vi "ROSServiceProvider.vi"(2 "Response":T2, 3 "ROS":T3={"topic port"=1236, "Node"="/labview", "topic"="/robot/head/command_head_nod", "type"="std_msgs/Bool", "node port"=7000, "error "={"status"=FALSE, "code"=0, "source"=""}, "Direction"=enum."Publisher", "Update (ms)"=1, "FIFO size"=1}) -> ()   [LabVIEW 2015]
doc: "Opens new ports for services, updates services with master, and closes services"
uses:
  SubVIs/_ROSControl.ctl
  SubVIs/_ROSDirection.ctl
  Console/Servers/ServerSubs/MyState.ctl
  _ROSDefinition.vi
  MessageBuilding/std_msgs/subs/i16Scalar.vi
  MessageBuilding/std_msgs/subs/stringScalar.vi
panel:
  out "Queue":string
  out "Master Reply":T1(array[cluster])
  out "response":string
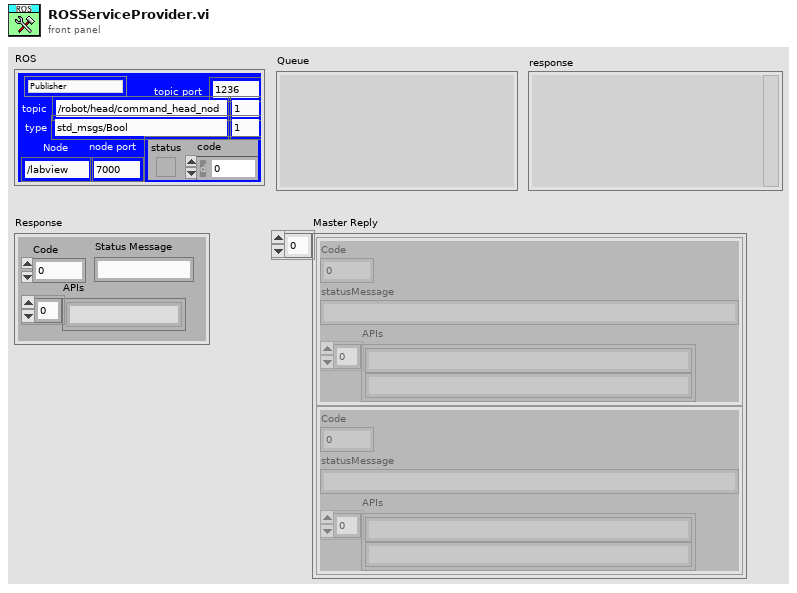
[diagram p1: front panel]
types:
  T1 = cluster{"Code":i8, "statusMessage":string, "APIs":string[]}[]
  T2 = cluster{"Code":i32, "Status Message":string, "APIs":string[]}
  T3 = typedef "_ROSControl.ctl" = cluster{"topic port":u16, "Node":string, "topic":string, "type":string, "node port":u16, "error ":errorcluster, "Direction":T4, "Update (ms)":u16, "FIFO size":u16}
  T4 = typedef "_ROSDirection.ctl" = enum16{"Node", "Publisher", "Subscriber", "ServiceClient", "ServiceProvider"}
  T5 = typedef "MyState.ctl" = enum16{"No Connection", "Registered", "Connected", "Close"}
  T6 = enum16{"Reset Log", "Add Client", "Remove Client", "Add Task"}
  T7 = typedef "ROSLog.ctl" = cluster{"Sent":string, "Reply":string, "MethodName":string, "success":bool, "Dir1":string, "Dir2":string, "Time Stamp":string, "error":errorcluster, "Preamble":string, "Midamble":string, "Postamble":string}
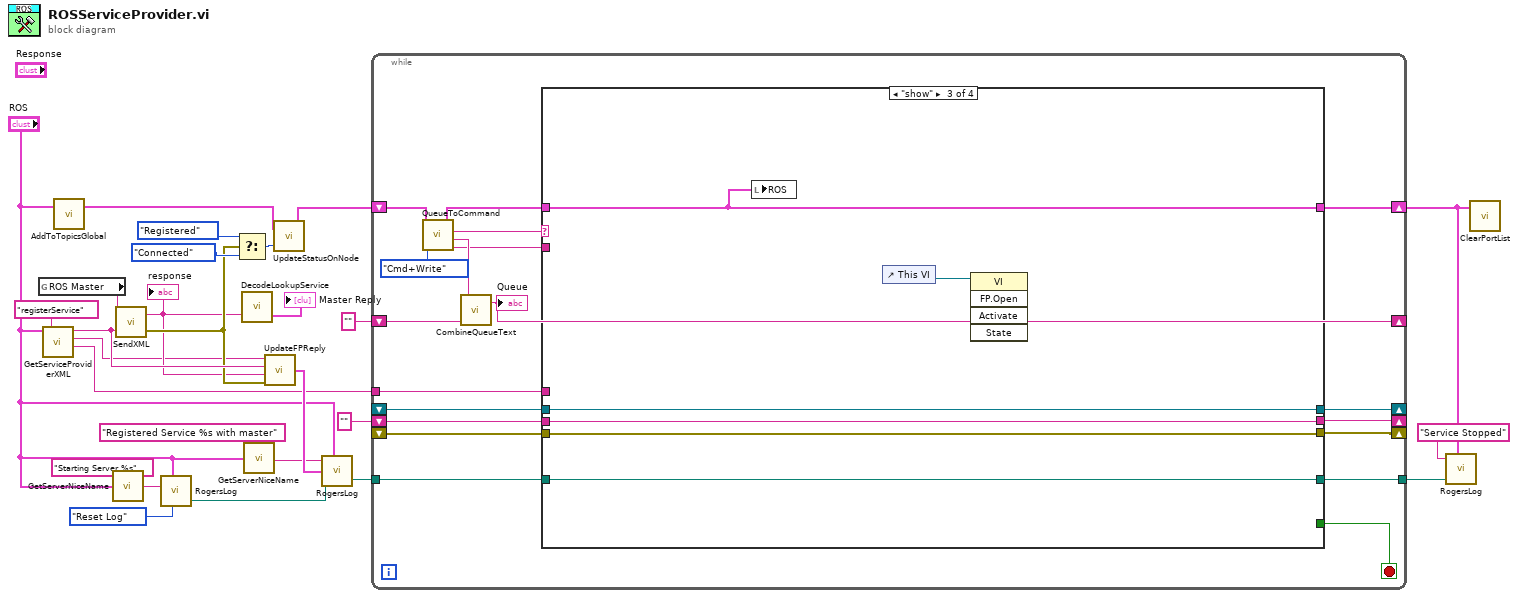
[diagram p0: block diagram]
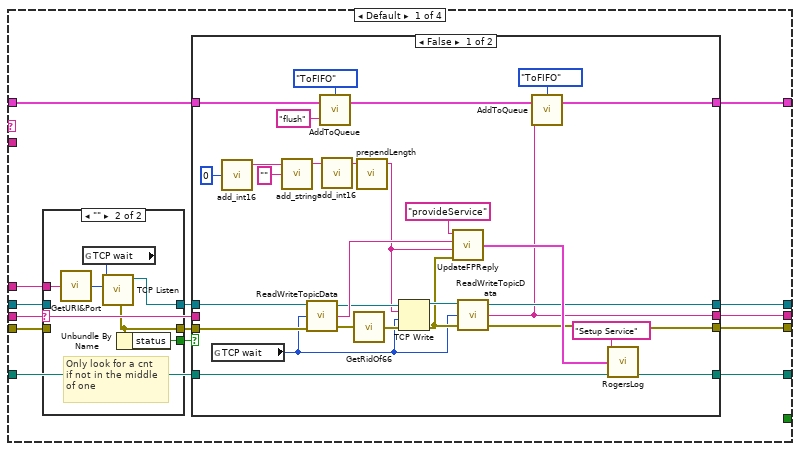
[diagram p2: hidden frame]
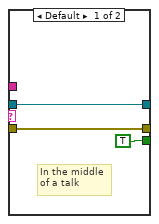
[diagram p3: hidden frame]
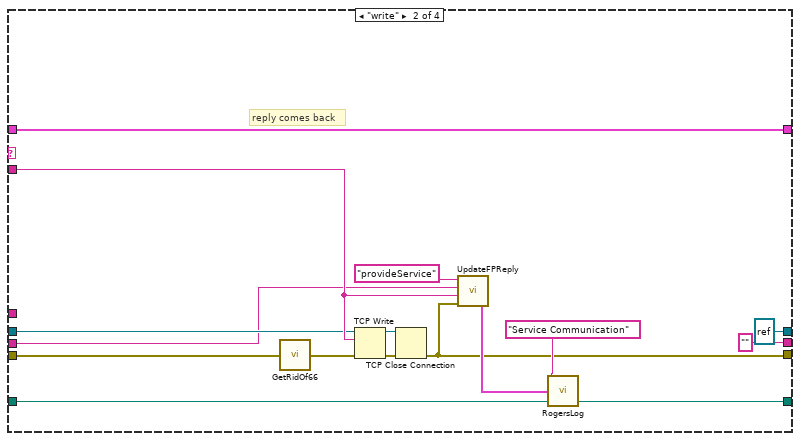
[diagram p5: hidden frame]
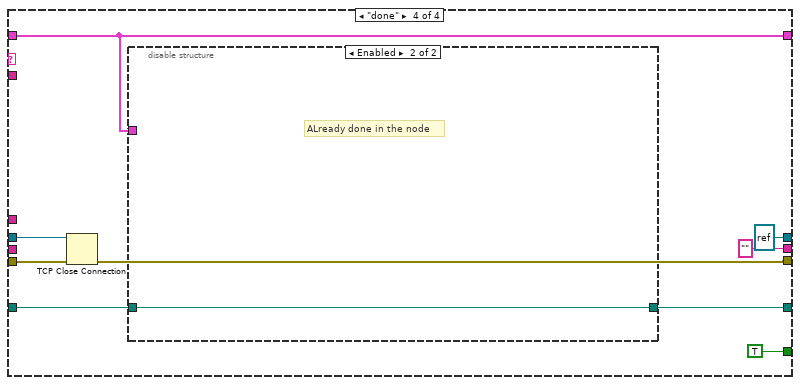
[diagram p6: hidden frame]
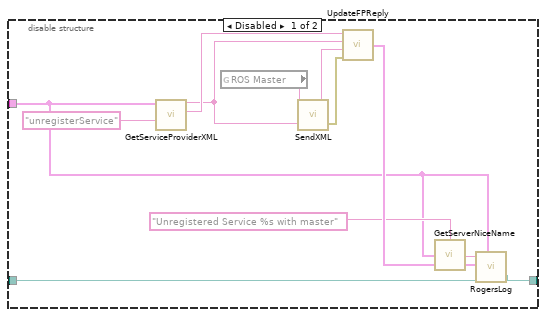
[diagram p7: hidden frame]
diagram:
  n1 = global read "_ROSDefinition.vi" "ROS Master"() -> (w23:string)
  n2 = call "GetServiceProviderXML.vi"("Method Name"="registerService", "ROS"="ROS") -> ("URI"=w6:string, "Method Name"=w9:string, "lookupService"=w24:string)  [unwired: 7 in]
  n3 = call "AddToTopicsGlobal.vi"("ROS in"="ROS") -> ("ROS out"=w3:T3)  [unwired: 2 in]
  n4 = call "GetServerNiceName.vi"("ROS"="ROS", "Text to add"="Starting Server %s") -> ("String"=w26:string)
  n5 = call "SendXML.vi"("Send"=w24, "URI in"=w23) -> ("error out"=w15:errorcluster, "Reply"=w14:string)
  "response" <- w14
  n6 = call "RogersLog.vi"("Text to add"=w26, "ROS"="ROS", "Task"=T6."Reset Log") -> ("LogPath out"=w18:path)  [unwired: 2 in, 1 out]
  n7 = Select(t=MyState."Registered" ("MyState"), s=w15, f=MyState."Connected" ("MyState")) -> (s? t:f=w20:T5)
  n8 = call "DecodeLookupService.vi"("Response"=w14) -> ("Reply"=→"Master Reply":T1)  [unwired: 2 in]
  n9 = call "GetServerNiceName.vi"("ROS"="ROS", "Text to add"="Registered Service %s with master") -> ("String"=w16:string)
  n10 = call "UpdateFPReply.vi"("error in (no error)"=w15, "Reply"=w14, "Sent"=w24, "method"=w9) -> ("Log"=w19:T7)
  n11 = call "UpdateStatusOnNode.vi"("MyState"=w20, "ROS"=w3) -> ("ROS out"=w2:T3)  [unwired: 1 in]
  n12 = call "RogersLog.vi"("Text to add"=w16, "ROS"="ROS", "Log"=w19, "LogPath in"=w18) -> ("LogPath out"=w11:path)  [unwired: 1 in, 1 out]
  n13 = while {
    tunnel: w11 -> [w46]
    tunnel: [w45] -> w10
    shift-right: [w41] -> _
    shift-left: "" ("New List") -> [w42]
    tunnel: w6 -> [w40]
    shift-right: [w36] -> _
    shift-left: _ -> [w33]
    shift-right: [w35] -> _
    shift-left: "" ("data out") -> [w31]
    shift-right: [w34] -> _
    shift-left: _ -> [w32]
    shift-right: [w29] -> w1
    shift-left: w2 -> [w39]
    stop <- w44 stop-if-true
    n14 = call "QueueToCommand.vi"("ROS"=w39, "Check"=enum16{"Cmd+Write", "FIFO", "CMD", "CMD /wait"}."Cmd+Write") -> ("ROS out"=w30:T3, "Command"=w38:string, "Queue log"=w43:string, "data"=w37:string)  [unwired: 1 in]
    n15 = call "CombineQueueText.vi"("Old List"=w42, "Queue In"=w43) -> ("New List"=w41:string)  [unwired: 1 in]
    "Queue" <- w41
    n16 = case shown="\"show\"" w38 {
      tunnel: w30 -> [w59 w106 w120 w133]
      tunnel: w46 -> [w58 w109 w125 w132]
      tunnel: [w57 w108 w125 w131] -> w45
      tunnel: w37 -> [_ w114 _ _]
      tunnel: [w47 w106 w120 w133] -> w29
      tunnel: [_ _ _ TRUE] -> w44
      tunnel: w40 -> [w56 _ _ _]
      tunnel: [w55 refnum<k5> refnum ("connection ID out") w121 refnum<k5> refnum ("connection ID out")] -> w36
      tunnel: [w54 "" ("data out") w122 "" ("data out")] -> w35
      tunnel: [w53 w107 w123 w128] -> w34
      tunnel: w33 -> [w50 w112 w121 w129]
      tunnel: w32 -> [w51 w111 w123 w130]
      tunnel: w31 -> [w52 w110 w122 _]
      frame Default {
        n17 = case shown="\"\"" w52 {
          tunnel: [w63 w65] -> w49
          tunnel: [w62 w68] -> w60
          tunnel: w56 -> [_ w66]
          tunnel: w51 -> [w63 _]
          tunnel: w50 -> [w62 _]
          tunnel: [TRUE w64] -> w48
          frame Default {
            # "In the middle\nof a talk"
          }
          frame "" {
            # "Only look for a cnt\nif not in the middle\nof one"
            n18 = call "GetURI&Port.vi"("URI in"=w66) -> ("Port"=w69:u16)  [unwired: 1 out]
            n19 = global read "_ROSDefinition.vi" "TCP wait"() -> (w67:i32)
            n20 = call "TCP Listen.vi"("timeout ms (wait forever: -1)"=w67, "port"=w69) -> ("error out"=w65:errorcluster, "connection ID"=w68:refnum<k5>)  [unwired: 5 in, 3 out]
            n21 = Unbundle By Name(w65) -> ("status"=w64:bool)
          }
        }
        n22 = case shown="False" w48 {
          tunnel: w60 -> [w98 w102]
          tunnel: w58 -> [w94 w103]
          tunnel: w59 -> [w73 w99]
          tunnel: [w77 w103] -> w57
          tunnel: [w80 w102] -> w55
          tunnel: [w79 w101] -> w54
          tunnel: [w78 w100] -> w53
          tunnel: w52 -> [_ w101]
          tunnel: w49 -> [w76 w100]
          tunnel: [w71 w99] -> w47
          frame False {
            n23 = global read "_ROSDefinition.vi" "TCP wait"() -> (w75:i32)
            n24 = call-poly "add_int16.vi"("Numeric"=i16 0) -> ("msg out"=w90:string)  [unwired: 4 in]
            n25 = call-poly "add_string.vi"("String"="", "msg in"=w90) -> ("msg out"=w91:string)  [unwired: 3 in]
            n26 = call "ReadWriteTopicData.vi"("error in (no error)"=w76, "timeout ms (1000)"=w75, "connection ID in"=w98) -> ("error out"=w97:errorcluster, "data out"=w96:string, "connection ID out"=w88:refnum<k5>)
            n27 = call "AddToQueue.vi"("Cmd"="flush", "ROS"=w73, "Type"=enum16{"topic", "node", "ToFIFO", "ToWrite"}."ToFIFO") -> ("ROS out"=w72:T3)  [unwired: 2 in]
            n28 = call-poly "add_int16.vi"("msg in"=w91) -> ("msg out"=w83:string)  [unwired: 4 in]
            n29 = call "GetRidOf66.vi"("error in (no error)"=w97) -> ("error out"=w89:errorcluster)
            n30 = call "prependLength.vi"("msg in"=w83) -> ("msg out"=w82:string)  [unwired: 4 in]
            n31 = TCP Write(connection ID=w88, data in=w82, error in (no error)=w89, 9:w75) -> (connection ID out=w87:refnum<k5>, error out=w86:errorcluster)  [unwired: 1 out]
            n32 = call "UpdateFPReply.vi"("error in (no error)"=w86, "Reply"=w82, "Sent"=w96, "method"="provideService") -> ("Log"=w85:T7)
            n33 = call "ReadWriteTopicData.vi"("error in (no error)"=w86, "timeout ms (1000)"=w75, "connection ID in"=w87) -> ("error out"=w78:errorcluster, "data out"=w79:string, "connection ID out"=w80:refnum<k5>)
            n34 = call "AddToQueue.vi"("Cmd"=w79, "ROS"=w72, "Type"=enum16{"topic", "node", "ToFIFO"}."ToFIFO") -> ("ROS out"=w71:T3)  [unwired: 2 in]
            n35 = call "RogersLog.vi"("Text to add"="Setup Service", "Log"=w85, "LogPath in"=w94) -> ("LogPath out"=w77:path)  [unwired: 2 in, 1 out]
          }
          frame True {
          }
        }
      }
      frame "write" {
        # "reply comes back"
        n36 = call "GetRidOf66.vi"("error in (no error)"=w111) -> ("error out"=w119:errorcluster)
        n37 = TCP Write(connection ID=w112, data in=w114, error in (no error)=w119) -> (connection ID out=w117:refnum<k5>, error out=w118:errorcluster)  [unwired: 1 in, 1 out]
        n38 = TCP Close Connection(connection ID=w117, error in (no error)=w118) -> (error out=w107:errorcluster)  [unwired: 1 in, 1 out]
        n39 = call "UpdateFPReply.vi"("error in (no error)"=w107, "Reply"=w114, "Sent"=w110, "method"="provideService") -> ("Log"=w115:T7)
        n40 = call "RogersLog.vi"("Text to add"="Service Communication", "Log"=w115, "LogPath in"=w109) -> ("LogPath out"=w108:path)  [unwired: 2 in, 1 out]
      }
      frame "show" {
        n41 = local write "ROS"(w120) -> ()
        n42 = control-ref of="This VI"() -> (w124:refnum<vi>)
        n43 = invoke class="VI" method="FP.Open"(reference=w124) -> ()  [unwired: 4 in, 5 out]
      }
      frame "done" {
        n44 = TCP Close Connection(connection ID=w129, error in (no error)=w130) -> (error out=w128:errorcluster)  [unwired: 1 in, 1 out]
        n45 = disable-structure shown="Enabled" {
          disable-tunnel: w133 -> [w138 _]
          disable-tunnel: w132 -> [w136 w147]
          disable-tunnel: [w135 w147] -> w131
          frame Disabled {
            n46 = call "GetServiceProviderXML.vi"("Method Name"="unregisterService", "ROS"=w138) -> ("Method Name"=w143:string, "lookupService"=w142:string)  [unwired: 7 in, 1 out]
            n47 = global read "_ROSDefinition.vi" "ROS Master"() -> (w146:string)
            n48 = call "SendXML.vi"("Send"=w142, "URI in"=w146) -> ("error out"=w144:errorcluster, "Reply"=w141:string)
            n49 = call "UpdateFPReply.vi"("error in (no error)"=w144, "Reply"=w141, "Sent"=w142, "method"=w143) -> ("Log"=w140:T7)
            n50 = call "GetServerNiceName.vi"("ROS"=w138, "Text to add"="Unregistered Service %s with master") -> ("String"=w137:string)
            n51 = call "RogersLog.vi"("Text to add"=w137, "ROS"=w138, "Log"=w140, "LogPath in"=w136) -> ("LogPath out"=w135:path)  [unwired: 1 in, 1 out]
          }
          frame Enabled {
            # "ALready done in the node"
          }
        }
      }
    }
  }
  n52 = call "RogersLog.vi"("Text to add"="Service Stopped", "ROS"=w1, "LogPath in"=w10) -> ()  [unwired: 2 in, 2 out]
  n53 = call "ClearPortList.vi"("ROS"=w1) -> ()  [unwired: 2 in]
